vi "Load Glyph.vi"(8 "error in (no error)":errorcluster, 10 "Path":path, 11 "PictureBox in":refnum<k24>) -> (0 "error out":errorcluster, 3 "PictureBox out":refnum<k24>)   [LabVIEW 2019, in "Configuration Tool.lvlib"]
uses:
  Configuration Tool.lvlib
  System.Windows.Forms
  System.Drawing
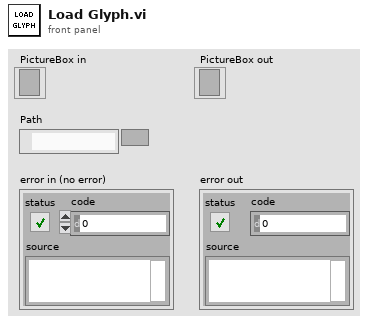
[diagram p1: front panel]
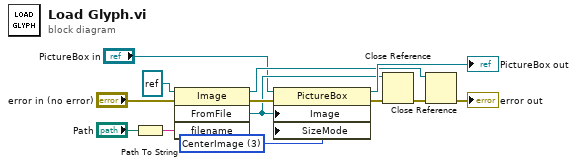
[diagram p0: block diagram]
diagram:
  w1 = 3 items=["Normal", "StretchImage", "AutoSize", "CenterImage", "Zoom"] ("SizeMode")
  n1 = Path To String(path="Path") -> (string=w12:string)
  n2 = invoke class="Image" method="FromFile"(reference=refnum<k24> refnum ("Image"), error in="error in (no error)", "filename"=w12) -> (reference out=w4:refnum<k24>, error out=w10:errorcluster, "FromFile"=w6:refnum<k24>)  [unwired: 1 in, 1 out]
  n3 = property class="PictureBox"(reference="PictureBox in", error in=w10, "Image"=w6, "SizeMode"=w1) -> (reference out=→"PictureBox out":refnum<k24>, error out=w8:errorcluster)
  n4 = Close Reference(reference=w6, error in (no error)=w8) -> (error out=w5:errorcluster)
  n5 = Close Reference(reference=w4, error in (no error)=w5) -> (error out=→"error out":errorcluster)
